vi "Get Attributes.vi"(8 "error in (no error)":errorcluster, 11 "For Loop Dialog in":refnum<class "Name Only Dialog.lvclass">) -> (0 "error out":errorcluster, 3 "For Loop Dialog out":refnum<class "Name Only Dialog.lvclass">)   [LabVIEW 2017, in "Name Only Dialog.lvclass"]
uses:
  Name Only Dialog.lvclass
  ITest Executive Builder Dialog/ITest Executive Builder Dialog.lvclass
  <vilib>/gpm_packages/@cs/test-executive/Source/Test Executive/TestExecutive Ref/TestExecutive Ref.lvclass
  C:/Users/huijun.guo/Desktop/composed-test-executive-builder/Source/Test Executive Builder Dialogs/ITest Executive Builder Dialog/ITest Executive Builder Dialog.lvclass
  C:/Program Files/National Instruments/LabVIEW 2017/vi.lib/gpm_packages/@cs/popup-viewmanager/Source/Popup ViewManager/Popup ViewManager.lvclass
  C:/Program Files/National Instruments/LabVIEW 2017/vi.lib/gpm_packages/@cs/mva-dialogbox/source/IDialogBox/IDialogBox/IDialogBox.lvclass
  C:/Program Files/National Instruments/LabVIEW 2017/vi.lib/gpm_packages/@cs/mva-viewable/Source/IViewable/IViewable/IViewable.lvclass
  C:/Program Files/National Instruments/LabVIEW 2017/vi.lib/gpm_packages/@cs/mva-viewable/Source/ActorEvents/IEventAggregator/IEventAggregator.lvclass
  C:/Program Files/National Instruments/LabVIEW 2017/vi.lib/gpm_packages/@cs/mva-core/Source/IObserver/IObserver/IObserver.lvclass
  C:/Program Files/National Instruments/LabVIEW 2017/vi.lib/ActorFramework/Actor/Actor.lvclass
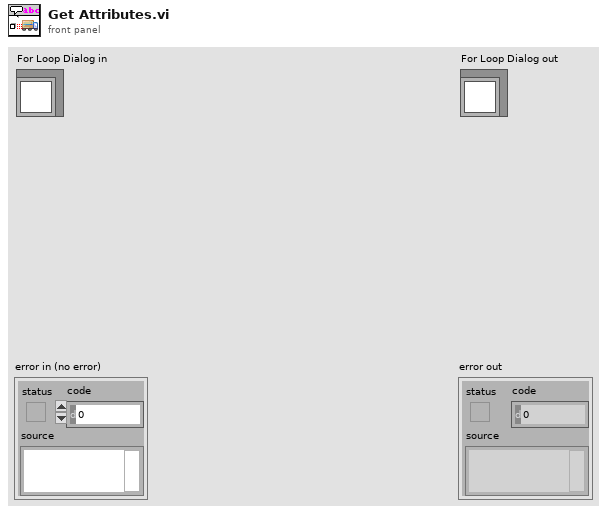
[diagram p1: front panel]
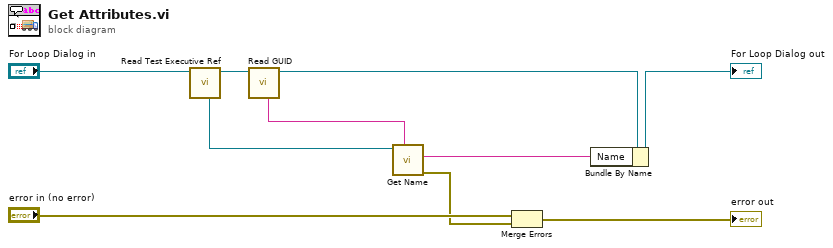
[diagram p0: block diagram]
diagram:
  n1 = call "Read Test Executive Ref.vi"("ITest Executive Builder Dialog in"="For Loop Dialog in") -> ("ITest Executive Builder Dialog out"=w9:refnum<class "Name Only Dialog.lvclass">, "Test Executive Ref"=w5:refnum<data-value>)  [unwired: 9 in]
  n2 = call "Read GUID.vi"("ITest Executive Builder Dialog in"=w9) -> ("ITest Executive Builder Dialog out"=w7:refnum<class "Name Only Dialog.lvclass">, "GUID"=w4:string)  [unwired: 9 in]
  n3 = call <vilib>:"Get Name.vi"("Unique ID"=w4, "Test Executive Ref"=w5) -> ("error out"=w1:errorcluster, "Name"=w8:string)  [unwired: 5 in, 3 out]
  n4 = Merge Errors("error in (no error)", w1) -> (→"error out":errorcluster)
  n5 = Bundle By Name(cluster=w7, "Name"=w8) -> (→"For Loop Dialog out":refnum<class "Name Only Dialog.lvclass">)
